vi "Worked_Example_Trapazoidal_Rule.vi"() -> ()   [LabVIEW 2013]
panel:
  out "Approx. Integral":dbl=7.8845418102876925
  out "Waveform Graph":cluster{"Lower limit \"a\"":dbl, dbl, dbl[]}(graph)={"Lower limit \"a\""=0.0, 0.00042, array[10001 elements]}
  in  "Divisions \"N\"":dbl=10000.0
  in  "Upper limit \"b\"":dbl=4.2
  in  "Lower limit \"a\"":dbl
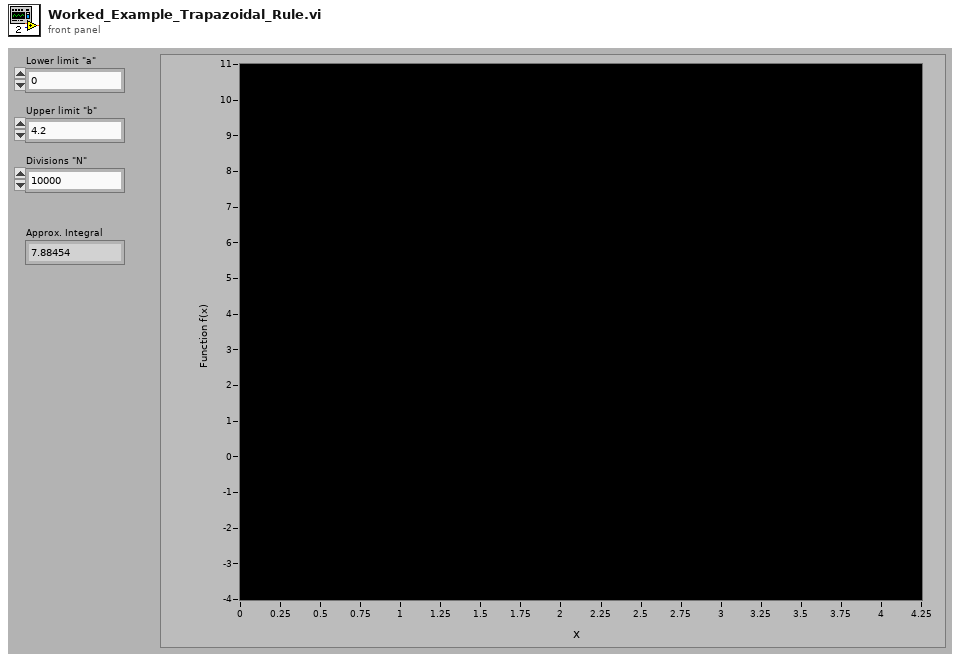
[diagram p1: front panel]
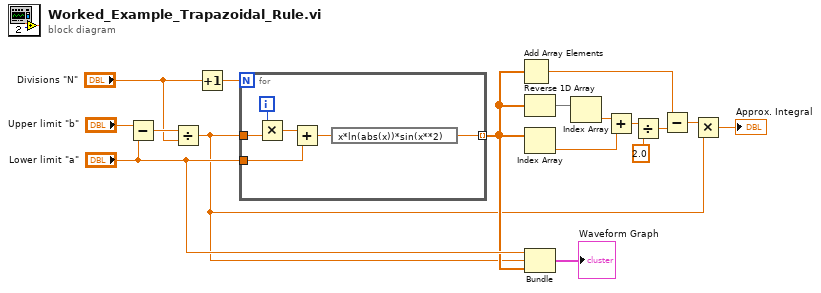
[diagram p0: block diagram]
diagram:
  n1 = Subtract(x="Upper limit \"b\"", y="Lower limit \"a\"") -> (x-y=w16:dbl)
  n2 = Divide(x=w16, y="Divisions \"N\"") -> (x/y=w2:dbl)
  n3 = Increment(x="Divisions \"N\"") -> (x+1=w14:dbl)
  n4 = for {
    N: w14 -> [_]
    tunnel: w2 -> [w22]
    tunnel: "Lower limit \"a\"" -> [w20]
    tunnel: [w19] -> w6 mode=indexing
    i -> [w23]
    n5 = Multiply(x=w23, y=w22) -> (x*y=w21:dbl)
    n6 = Add(x=w21, y=w20) -> (x+y=w18:dbl)
    n7 = expression code="x*ln(abs(x))*sin(x**2)"(w18) -> (w19:dbl)
  }
  n8 = Add Array Elements(numeric array=w6) -> (sum=w4:dbl)
  n9 = Reverse 1D Array(array=w6) -> (reversed array=w11:dbl[])
  n10 = Index Array(array=w6) -> (element=w9:dbl)  [unwired: 1 in]
  n11 = Bundle("Lower limit \"a\""="Lower limit \"a\"", w2, w6) -> (→"Waveform Graph":cluster{"Lower limit \"a\"":dbl, dbl, dbl[]})  [unwired: 1 in]
  n12 = Index Array(array=w11) -> (element=w10:dbl)  [unwired: 1 in]
  n13 = Add(x=w10, y=w9) -> (x+y=w8:dbl)
  n14 = Divide(x=w8, y=2.0) -> (x/y=w5:dbl)
  n15 = Subtract(x=w4, y=w5) -> (x-y=w3:dbl)
  n16 = Multiply(x=w3, y=w2) -> (x*y=→"Approx. Integral":dbl)
